vi "Is Variant LabVIEW Class.vi"(8 "Error In":errorcluster, 11 "Variant in":variant) -> (0 "Error Out":errorcluster, 3 "is variant LabVIEW class?":bool)   [LabVIEW 2014]
uses:
  <vilib>/Utility/VariantDataType/Type.ctl
  <vilib>/Utility/VariantDataType/VariantType.lvlib
panel:
  in  "LabVIEW Variant Data Types":T1
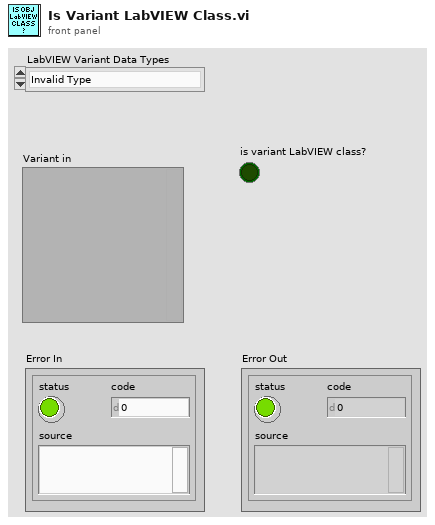
[diagram p1: front panel]
types:
  T1 = typedef "VariantType.lvlib/Type.ctl" = enum8{"Invalid Type", "Void", "I8", "I16", "I32", "I64", "U8", "U16", "U32", "U64", "Single Float", "Double Float", "Extended Float", "Single Complex", "Double Complex", "Extended Complex", "Enum U8", "Enum U16", "Enum U32", "Enum U64", "Single Float With Unit", "Double Float With Unit", "Extended Float With Unit", "Single Complex with Unit", "Double Complex with Unit", "Extended Complex with Unit", "Boolean", "String", "Path", "Picture", "Tag", "Array", "Cluster", "Variant", "LV Variant", "Waveform", "Timestamp", "Digital Waveform", "Digital Data", "ExpressData", "Refnum", "External Data", "VI", "Poly VI", "LabVIEW Class Instance", "Fixed Point"}
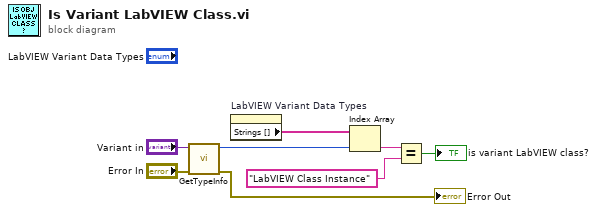
[diagram p0: block diagram]
diagram:
  n1 = call <vilib>:"GetTypeInfo.vi"("error in (no error)"="Error In", "Variant"="Variant in") -> ("error out"=→"Error Out":errorcluster, "Type Enum"=w8:T1)  [unwired: 5 in, 3 out]
  n2 = property on="LabVIEW Variant Data Types" class="Enum (strict)"() -> ("Strings []"=w1:string[])  [unwired: 2 in, 2 out]
  n3 = Index Array(array=w1, index=w8) -> (element=w6:string)
  n4 = Equal?(x=w6, y="LabVIEW Class Instance") -> (x = y?=→"is variant LabVIEW class?":bool)
